vi "Brower View Create.vi"(8 "error in (no error)":errorcluster, 11 "Brower View in":refnum<class "Brower View.lvclass">) -> (0 "error out":errorcluster, 3 "Brower View out":refnum<class "Brower View.lvclass">)   [LabVIEW 2015, in "Brower View.lvclass"]
uses:
  Brower View.lvclass
  Brower View.lvclass/Brower View.ctl
  MyTreeAPI/MyTreeAPI.lvclass
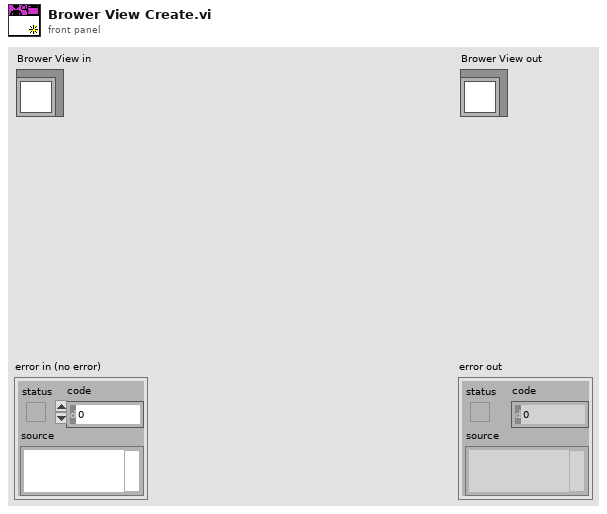
[diagram p1: front panel]
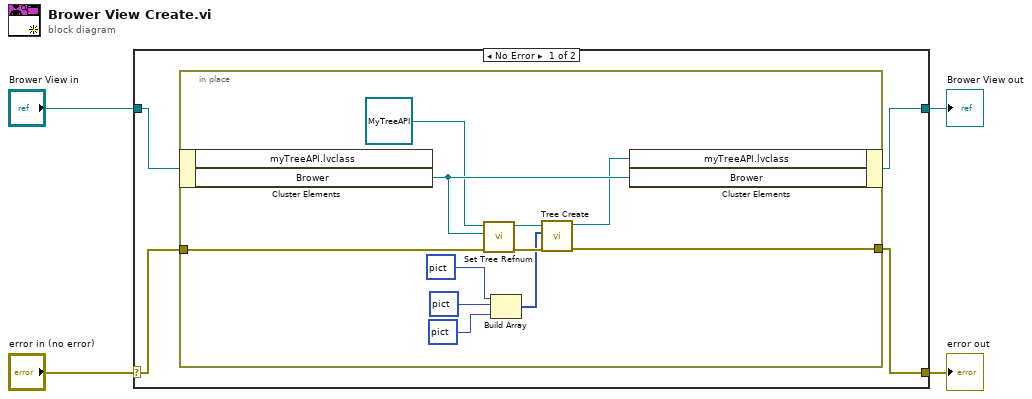
[diagram p0: block diagram]
diagram:
  n1 = case shown="No Error" "error in (no error)" {
    selector: "error in (no error)" -> [w7 w21]
    tunnel: [w6 w21] -> w3
    tunnel: [w5 w20] -> w1
    tunnel: "Brower View in" -> [w8 w20]
    frame No Error {
      n2 = in-place {
        in-place-border: w7 -> [w19]
        in-place-border: [w14] -> w6
        n3 = in-place-cluster #1(w8) -> ("Brower"=w18:refnum<vi>)  [unwired: 1 out]
        n4 = call "Set Tree Refnum.vi"("error in (no error)"=w19, "Tree"=w18, "TREE in"=refnum<class "MyTreeAPI.lvclass"> refnum) -> ("error out"=w13:errorcluster, "TREE out"=w16:refnum<class "MyTreeAPI.lvclass">)  [unwired: 7 in]
        n5 = Build Array(picture data[5B] ("2D Picture"), picture bytes[1570] ("2D Picture"), picture bytes[1570] ("2D Picture")) -> (w9:picture[])
        n6 = call "Tree Create.vi"("error in (no error)"=w13, "Symbols"=w9, "TREE in"=w16) -> ("error out"=w14:errorcluster, "TREE out"=w15:refnum<class "MyTreeAPI.lvclass">)  [unwired: 7 in]
        n7 = in-place-cluster #1("myTreeAPI.lvclass"=w15, "Brower"=w18) -> (w5:refnum<class "Brower View.lvclass">)
      }
    }
    frame Error {
    }
  }
  "error out" <- w3
  "Brower View out" <- w1
